vi "Read BombedWallParams.vi"(8 "error in (no error)":errorcluster, 11 "BombedWall":refnum<class "BombedWall.lvclass">) -> (0 "error out":errorcluster, 2 "BombedWallParams":T1, 3 "BombedWall":refnum<class "BombedWall.lvclass">)   [LabVIEW 2020, in "BombedWall.lvclass"]
uses:
  BombedWall.lvclass
  TypeDef/BombedWallParams.ctl
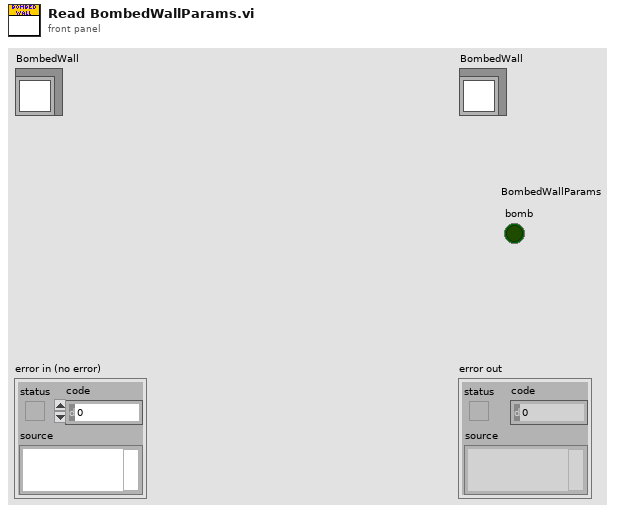
[diagram p1: front panel]
types:
  T1 = typedef "BombedWall.lvclass/BombedWallParams.ctl" = cluster{"bomb":bool}
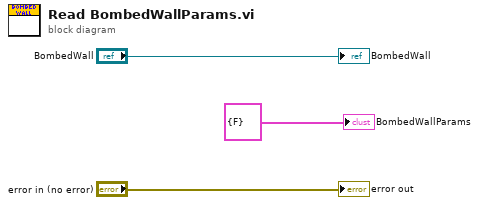
[diagram p0: block diagram]
diagram:
  "error out" <- "error in (no error)"
  "BombedWall" <- "BombedWall"
  "BombedWallParams" <- T1 {"bomb"=FALSE} ("<ClassName>Params")
